vi "adpm ap set minimum sync value.vi"(10 "minimum_sync_value":cluster{}, 11 "ap_handle":u32) -> (2 "function return":i32, 3 "ap_handle out":u32)   [LabVIEW 2019, in "apdm.lvlib"]
doc: "APDM_EXPORT int adpm_ap_set_minimum_sync_value(apdm_ap_handle_t ap_handle, const uint64_t minimum_sync_value);"
uses:
  apdm.lvlib
  Lee Lab/CP FES Walking 2018/Code/Working/LabVIEW/apdm.dll
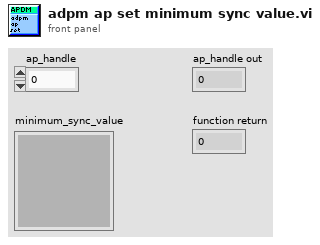
[diagram p1: front panel]
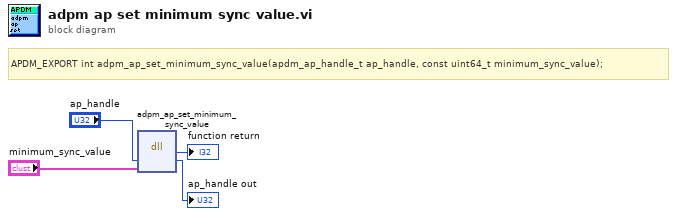
[diagram p0: block diagram]
diagram:
  # "APDM_EXPORT int adpm_ap_set_minimum_sync_value(apdm_ap_handle_t ap_handle, const uint64_t minimum_sync_value);"
  n1 = dll-call lib="C:/Users/jfalesi/Dropbox/Lee Lab/CP FES Walking 2018/Code/Working/LabVIEW/apdm.*" fn="adpm_ap_set_minimum_sync_value"("ap_handle"="ap_handle", "minimum_sync_value"="minimum_sync_value") -> (→"function return":i32, "ap_handle"=→"ap_handle out":u32)  [unwired: 4 in, 2 out]
